vi "Run.vi"(8 "error in (no error)":errorcluster, 9 "sprinkler data in":T2, 10 "Zone Setup Array":cluster{"Zone Selector":string, "Timing":dbl}[](array[cluster]), 11 "Controls":T3) -> (0 "error out":errorcluster, 2 "sprinkler data out":T2, 3 "state":T1)   [LabVIEW 2015]
uses:
  controls/sprinkler data.ctl
  controls/state.ctl
  controls/timerstatus.ctl
panel:
  # "Continuous"
  # "Single"
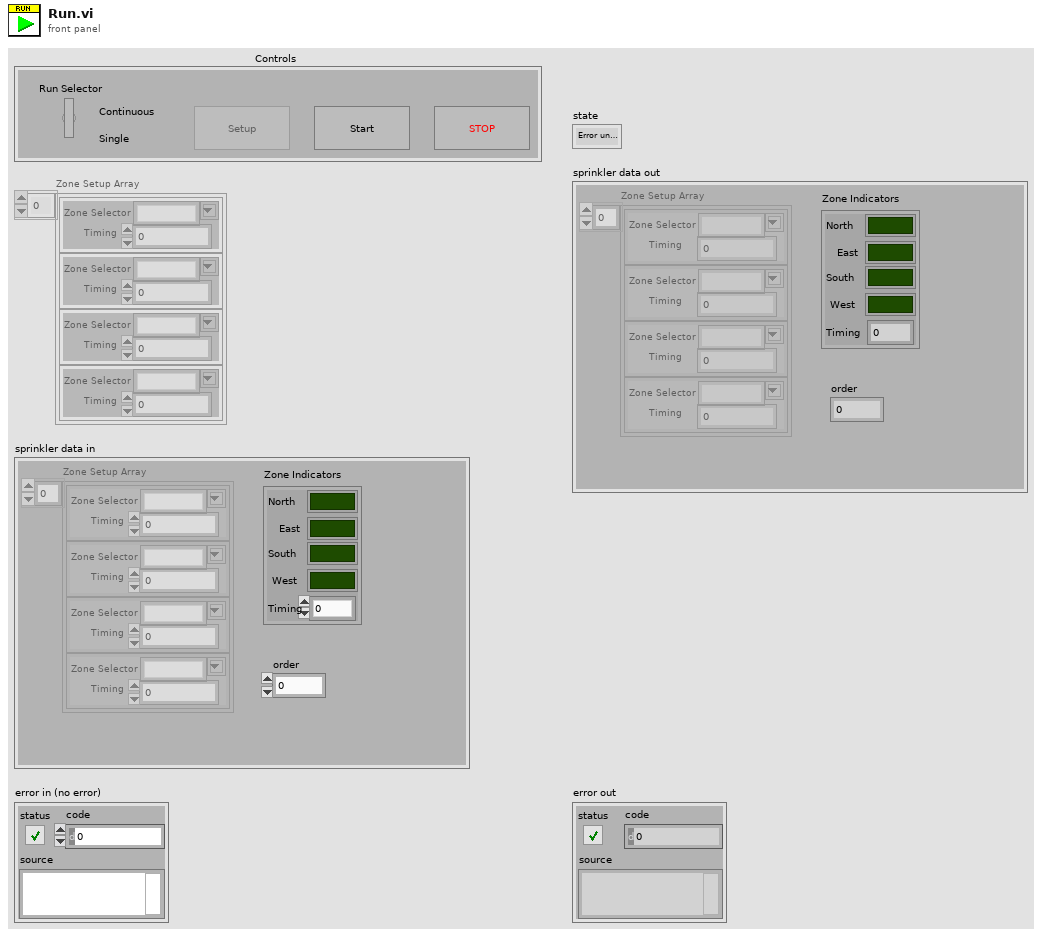
[diagram p1: front panel]
types:
  T1 = typedef "state.ctl" = enum16{"Error under range", "Exit", "Initialize", "Start", "Error", "Run", "Setup", "Low pressure", "Rain", "Idle"}
  T2 = typedef "sprinkler data.ctl" = cluster{"Zone Setup Array":cluster{"Zone Selector":string, "Timing":dbl}[], "Zone Indicators":cluster{"North":bool, "East":bool, "South":bool, "West":bool, "Timing":u32}, "order":i32}
  T3 = cluster{"Run Selector":bool, "Setup":bool, "Start":bool, "Stop":bool}
  T4 = typedef "timerstatus.ctl" = enum16{"Stop", "Start"}
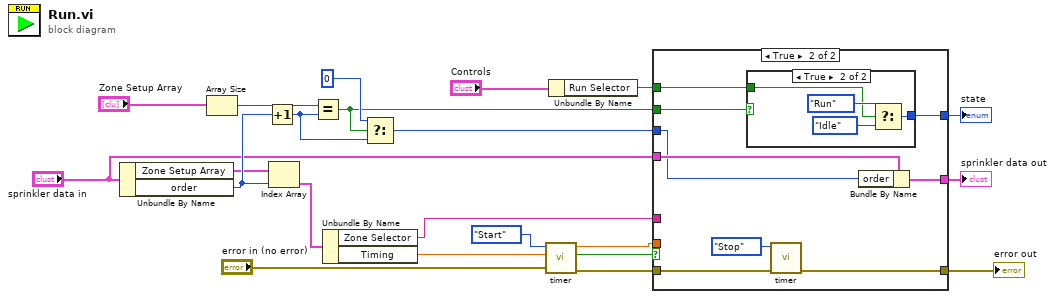
[diagram p0: block diagram]
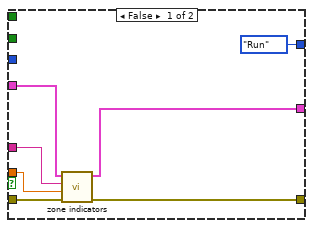
[diagram p2: hidden frame]
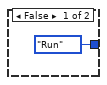
[diagram p3: hidden frame]
diagram:
  n1 = Unbundle By Name("sprinkler data in") -> ("Zone Setup Array"=w5:cluster{"Zone Selector":string, "Timing":dbl}[], "order"=w13:i32)
  n2 = Array Size(array="Zone Setup Array") -> (size(s)=w9:i32)
  n3 = Increment(x=w13) -> (x+1=w14:i32)
  n4 = Index Array(array=w5, index=w13) -> (element=w6:cluster{"Zone Selector":string, "Timing":dbl})
  n5 = Equal?(x=w9, y=w14) -> (x = y?=w1:bool)
  n6 = Unbundle By Name(w6) -> ("Zone Selector"=w2:string, "Timing"=w7:dbl)
  n7 = Select(t=0 ("order"), s=w1, f=w14) -> (s? t:f=w16:i32)
  n8 = call "timer.vi"("error in"="error in (no error)", "limit"=w7, "timerstat"=timerstatus."Start") -> ("error out"=w21:errorcluster, "in limit"=w11:bool, "elapsed"=w3:dbl)  [unwired: 6 in]
  n9 = Unbundle By Name("Controls") -> ("Run Selector"=w17:bool)
  n10 = case shown="True" w11 {
    tunnel: "sprinkler data in" -> [w24 w38]
    tunnel: w16 -> [_ w37]
    tunnel: w17 -> [_ w30]
    tunnel: [w23 w36] -> w18
    tunnel: [state."Run" ("f") w35] -> w19
    tunnel: w21 -> [w28 w34]
    tunnel: [w27 w33] -> w22
    tunnel: w3 -> [w26 _]
    tunnel: w2 -> [w25 _]
    tunnel: w1 -> [_ w31]
    frame False {
      n11 = call "zone indicators.vi"("error in (no error)"=w28, "Time"=w26, "Direction"=w25, "sprinkler data in"=w24) -> ("error out"=w27:errorcluster, "sprinkler data out"=w23:T2)  [unwired: 6 in]
    }
    frame True {
      n12 = case shown="True" w31 {
        tunnel: [state."Run" ("f") w42] -> w35
        tunnel: w30 -> [_ w40]
        frame False {
        }
        frame True {
          n13 = Select(t=state."Run" ("element"), s=w40, f=state."Idle") -> (s? t:f=w42:T1)
        }
      }
      n14 = call "timer.vi"("error in"=w34, "timerstat"=timerstatus."Stop") -> ("error out"=w33:errorcluster)  [unwired: 7 in, 2 out]
      n15 = Bundle By Name(cluster=w38, "order"=w37) -> (w36:T2)
    }
  }
  "sprinkler data out" <- w18
  "state" <- w19
  "error out" <- w22
